vi "VADC_TEST_SET.vi"(4 "itemiput":string, 5 "input":string, 6 "SEQ":i32, 7 "tpdata in":string[](array[string])) -> (3 "tpdata out":string[](array[string]))   [LabVIEW 2018]
panel:
  in  "高压机设置":bool
  in  "Standby Application":string
  in  "Bar":bool
  out "布尔":bool
  in  "退出":bool
  out "out":string
  in  "Tab Control":enum32{"DataSetign", "RelaySeting"}(tab)
  in  "Address":string(combo)="PCI-1713"
  in  "Start board number":string(combo)="1"
  in  "Test Type":string(combo)="0"
  in  "Output Current Max.Spec":string="*" caption="MAX"
  in  "Output Current Min.Spec":string="*" caption="MIN"
  in  "延时时间(ms)2":string="0" caption="Delay Time (ms)"
  in  "备注":string
  in  "H 2":bool[](array[boolean])
  in  "L 2":bool[](array[boolean])
  in  "H":bool[](array[boolean])
  in  "L":bool[](array[boolean])
  in  "L 3":bool[](array[boolean])
  in  "H 3":bool[](array[boolean])
  in  "L 4":bool[](array[boolean])
  in  "H 4":bool[](array[boolean])
  in  "Cancel":bool
  in  "OK":bool
  # "EditTestData"
  # "9-16位输出"
  # "1-8位输出"
  # "17-24位输出"
  # "25-32位输出"
  # "33-40位输出"
  # "41-48位输出"
  # "49-56位输出"
  # "57-64位输出"
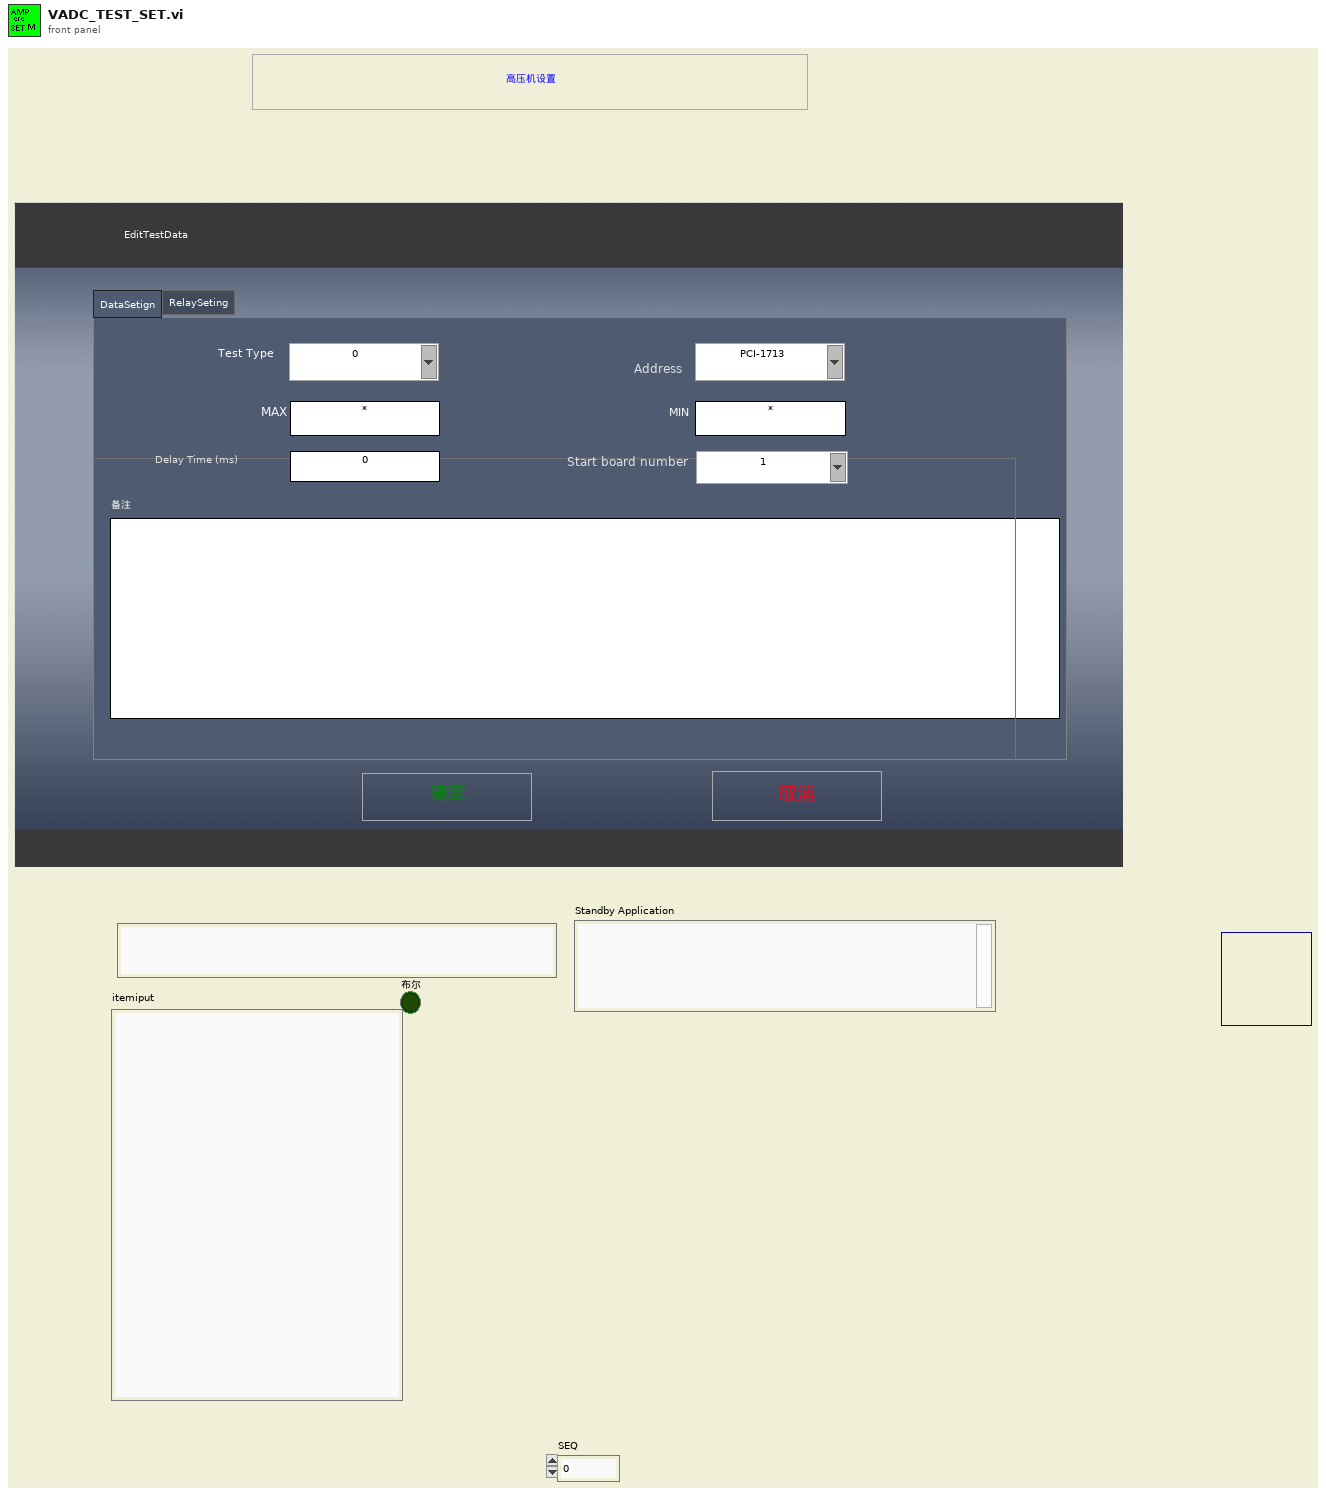
[diagram p1: front panel]
types:
  T1 = typedef "Window Refnum.ctl" = refnum<k1>
  T2 = typedef "Window Rectangle.ctl" = cluster{"left":i16, "top":i16, "right":i16, "bottom":i16}
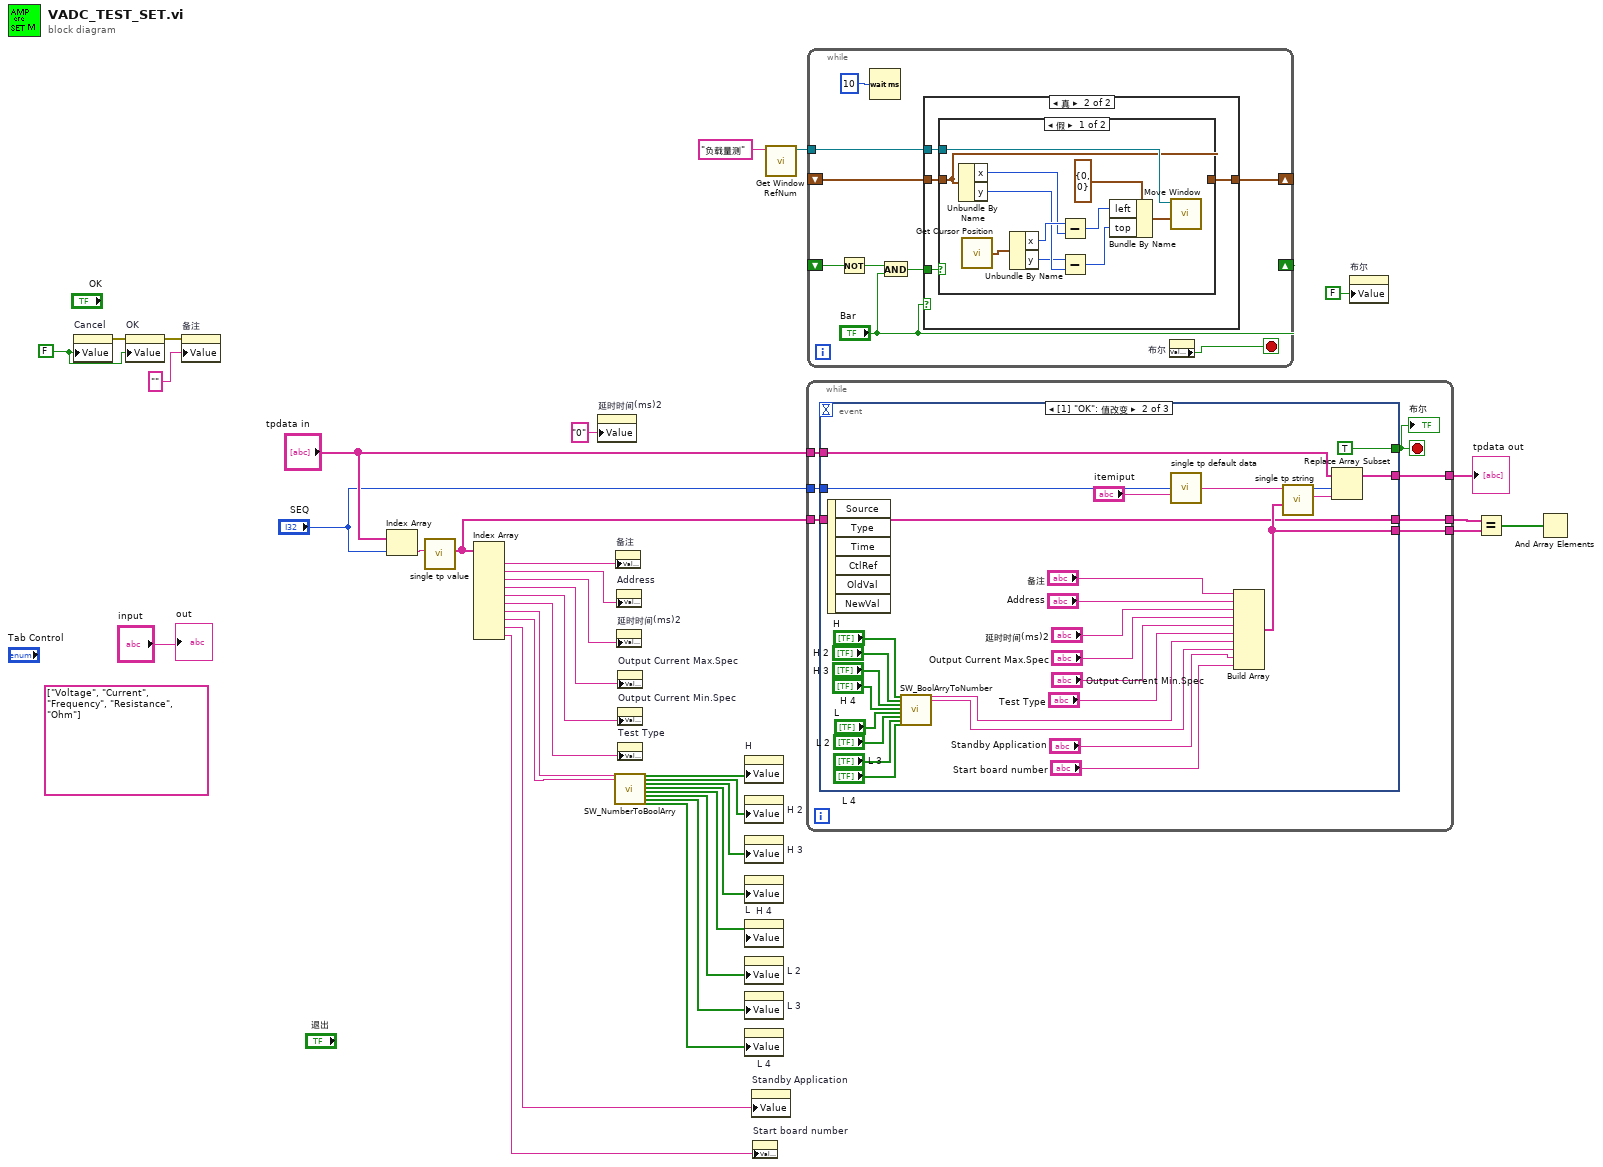
[diagram p0: block diagram]
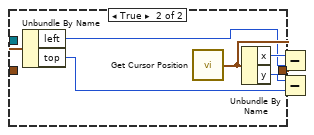
[diagram p3: hidden frame]
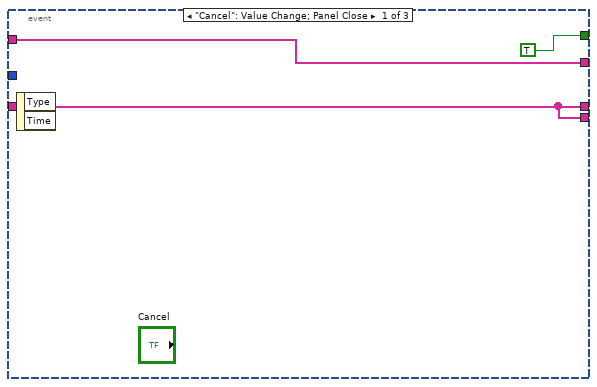
[diagram p4: hidden frame]
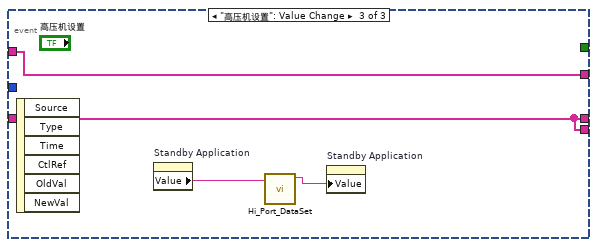
[diagram p5: hidden frame]
diagram:
  (unwired) string[] ["Voltage", "Current", "Frequency", "Resistance", "Ohm"]
  w32 = FALSE
  n1 = property on="Cancel" class="Bool (严格)"("Value"=w32) -> (error out=w34:errorcluster)  [unwired: 2 in, 1 out]
  n2 = property on="OK" class="Bool (严格)"(error in=w34, "Value"=w32) -> (error out=w33:errorcluster)  [unwired: 1 in, 1 out]
  n3 = property on="备注" class="Str"(error in=w33, "Value"="") -> ()  [unwired: 1 in, 2 out]
  n4 = Index Array(array="tpdata in", index="SEQ") -> (element=w22:string)
  n5 = call "single tp value.vi"("single tp data"=w22) -> ("value"=w20:string[])  [unwired: 10 out]
  n6 = Index Array(array=w20) -> (element #1=w21:string, element #2=w23:string, element #3=w24:string, element #4=w25:string, element #5=w26:string, element #6=w27:string, element #7=w13:string, element #8=w12:string, element #9=w1:string, element #10=w2:string)  [unwired: 10 in]
  n7 = property on="延时时间(ms)2" class="Str"("Value"="0" ("延时时间(ms)2")) -> ()  [unwired: 2 in, 2 out]
  n8 = call "SW_NumberToBoolArry.vi"("L STR"=w13, "H STR"=w12) -> ("H1"=w11:bool[], "H2"=w10:bool[], "H3"=w9:bool[], "H4"=w8:bool[], "L1"=w7:bool[], "L2"=w6:bool[], "L3"=w5:bool[], "L4"=w4:bool[])  [unwired: 18 in]
  n9 = property on="备注" class="Str"("Value"=w21) -> ()  [unwired: 2 in, 2 out]
  n10 = property on="Address" class="CmbBox"("Value"=w23) -> ()  [unwired: 2 in, 2 out]
  n11 = property on="延时时间(ms)2" class="Str"("Value"=w24) -> ()  [unwired: 2 in, 2 out]
  n12 = property on="Output Current Max.Spec" class="Str"("Value"=w25) -> ()  [unwired: 2 in, 2 out]
  n13 = property on="Output Current Min.Spec" class="Str"("Value"=w26) -> ()  [unwired: 2 in, 2 out]
  n14 = property on="Test Type" class="CmbBox"("Value"=w27) -> ()  [unwired: 2 in, 2 out]
  n15 = property on="H" class="Arr (严格)"("Value"=w11) -> ()  [unwired: 2 in, 2 out]
  n16 = property on="H 2" class="Arr (严格)"("Value"=w10) -> ()  [unwired: 2 in, 2 out]
  n17 = property on="H 3" class="Arr (严格)"("Value"=w9) -> ()  [unwired: 2 in, 2 out]
  n18 = property on="H 4" class="Arr (严格)"("Value"=w8) -> ()  [unwired: 2 in, 2 out]
  n19 = property on="L" class="Arr (严格)"("Value"=w7) -> ()  [unwired: 2 in, 2 out]
  n20 = property on="L 2" class="Arr (严格)"("Value"=w6) -> ()  [unwired: 2 in, 2 out]
  n21 = property on="L 3" class="Arr (严格)"("Value"=w5) -> ()  [unwired: 2 in, 2 out]
  n22 = property on="L 4" class="Arr (严格)"("Value"=w4) -> ()  [unwired: 2 in, 2 out]
  n23 = property on="Standby Application" class="Str"("Value"=w1) -> ()  [unwired: 2 in, 2 out]
  n24 = property on="Start board number" class="CmbBox"("Value"=w2) -> ()  [unwired: 2 in, 2 out]
  n25 = call "Get Window RefNum.vi"("window name (\"\")"="负载量测" ("window name (\"\")")) -> ("window refnum (NaWR)"=w15:T1)  [unwired: 1 in, 7 out]
  n26 = while {
    tunnel: "tpdata in" -> [w41]
    tunnel: [w40] -> w29
    tunnel: "SEQ" -> [w39]
    tunnel: [w38] -> w28
    tunnel: w20 -> [w37]
    tunnel: [w36] -> w31
    stop <- w42 stop-if-true
    n27 = event shown="[1] \"OK\": 值改变" {
      selector: _ -> [_ _ _]
      dyn-events: _ -> [_ _ _]
      timeout: _ -> [_ _ _]
      tunnel: [TRUE TRUE _] -> w42
      tunnel: [w44 w68 w76] -> w40
      tunnel: w41 -> [w44 w69 w76]
      tunnel: w39 -> [_ w67 _]
      tunnel: [w43 w65 w75] -> w38
      tunnel: w37 -> [w43 w64 w75]
      tunnel: [w43 w64 w75] -> w36
      event "Cancel": Value Change; Panel Close {
        n28 = event-data() -> ()  [unwired: 3 out]
      }
      event "OK": Value Change {
        n29 = event-data() -> ()  [unwired: 7 out]
        n30 = call "SW_BoolArryToNumber.vi"("L1"="H", "L 2"="H 2", "L 3"="H 3", "L 4"="H 4", "L 5"="L", "L 6"="L 2", "L 7"="L 3", "L 8"="L 4") -> ("H"=w48:string, "L"=w49:string)  [unwired: 18 in]
        n31 = call "single tp default data.vi"("字符串"="itemiput") -> ("item data"=w71:string)
        n32 = Build Array("备注", "Address", "延时时间(ms)2", "Output Current Max.Spec", "Output Current Min.Spec", "Test Type", w48, w49, "Standby Application", "Start board number") -> (w65:string[])
        n33 = call "single tp string.vi"("value in"=w65, "oringnal defult tp data"=w71) -> ("new single tp data out"=w70:string)  [unwired: 9 out]
        n34 = Replace Array Subset(array=w69, new element=w70, index=w67) -> (w68:string[])
      }
      event "高压机设置": Value Change {
        n35 = event-data() -> ()  [unwired: 7 out]
        n36 = property on="Standby Application" class="Str"() -> ("Value"=w73:string)  [unwired: 2 in, 2 out]
        n37 = call "Hi_Port_DataSet.vi"("InputStr"=w73) -> ("OutStr"=w74:string)  [unwired: 10 in]
        n38 = property on="Standby Application" class="Str"("Value"=w74) -> ()  [unwired: 2 in, 2 out]
      }
    }
    "布尔" <- w42
  }
  "tpdata out" <- w29
  n39 = while {
    shift-left: _ -> [w79]
    shift-right: [w80] -> _
    shift-left: _ -> [w83]
    shift-right: ["Bar"] -> _
    tunnel: w15 -> [w84]
    stop <- w77 stop-if-true
    n40 = Not(x=w83) -> (.not. x?=w82:bool)
    n41 = Wait (ms)(milliseconds to wait=u32 10) -> ()  [unwired: 1 out]
    n42 = And(x=w82, y="Bar") -> (x .and. y?=w78:bool)
    n43 = case shown="真" "Bar" {
      tunnel: w84 -> [_ w90]
      tunnel: [w86 w89] -> w80
      tunnel: w79 -> [w86 w87]
      tunnel: w78 -> [_ w88]
      frame False {
      }
      frame True {
        n44 = case shown="假" w88 {
          tunnel: w90 -> [w96 w112]
          tunnel: [w91 w102] -> w89
          tunnel: w87 -> [w91 _]
          frame False {
            n45 = Unbundle By Name(w91) -> ("x"=w99:i16, "y"=w98:i16)
            n46 = call "Get Cursor Position.vi"() -> ("cursor position"=w101:cluster{"x":i16, "y":i16})
            n47 = Unbundle By Name(w101) -> ("x"=w100:i16, "y"=w97:i16)
            n48 = Subtract(x=w100, y=w99) -> (x-y=w93:i16)
            n49 = Subtract(x=w97, y=w98) -> (x-y=w94:i16)
            n50 = Bundle By Name(cluster=cluster{"left":i16, "top":i16} {"left"=0, "top"=0} ("new position (0,0)"), "left"=w93, "top"=w94) -> (w92:cluster{"left":i16, "top":i16})
            n51 = call "Move Window.vi"("new position (0,0)"=w92, "window refnum (NaWR)"=w96) -> ()  [unwired: 2 in, 4 out]
          }
          frame True {
            n52 = call "Get Window Rectangle.vi"("window refnum (NaWR)"=w112) -> ("window rect"=w111:T2)  [unwired: 1 in, 5 out]
            n53 = call "Extract Window Origin.vi"("window rect"=w111) -> ("window origin"=w110:cluster{"left":i16, "top":i16})  [unwired: 1 out]
            n54 = Unbundle By Name(w110) -> ("left"=w107:i16, "top"=w106:i16)
            n55 = call "Get Cursor Position.vi"() -> ("cursor position"=w109:cluster{"x":i16, "y":i16})
            n56 = Unbundle By Name(w109) -> ("x"=w108:i16, "y"=w105:i16)
            n57 = Subtract(x=w108, y=w107) -> (x-y=w103:i16)
            n58 = Subtract(x=w105, y=w106) -> (x-y=w104:i16)
            n59 = Bundle By Name(cluster=w109, "x"=w103, "y"=w104) -> (w102:cluster{"x":i16, "y":i16})
          }
        }
      }
    }
    n60 = property on="布尔" class="Bool (严格)"() -> ("Value"=w77:bool)  [unwired: 2 in, 2 out]
  }
  n61 = property on="布尔" class="Bool (严格)"("Value"=FALSE ("布尔")) -> ()  [unwired: 2 in, 2 out]
  n62 = Equal?(x=w31, y=w28) -> (x = y?=w30:bool[])
  n63 = And Array Elements(Boolean array=w30) -> ()  [unwired: 1 out]
  "out" <- "input"
